vi "Dashboard Main.vi"() -> ()   [LabVIEW 2012]
uses:
  <vilib>/event_ctls.llb/eventvkey.ctl
  <vilib>/Utility/config.llb/Read Key (String).vi
  <vilib>/Utility/config.llb/Read Key (I32).vi
  <vilib>/Utility/config.llb/Write Key (String).vi
  <vilib>/Utility/config.llb/Write Key (I32).vi
  <vilib>/Utility/config.llb/NI_LVConfig.lvlib
panel:
  out "Battery Value":dbl(slide) scale=0.0..14.0 scale format="%#_2e"
  out "Battery":sgl(graph)
  in  "Camera Settings":T1={"Frate Rate"=30, "Compression"=30, "Size"=1} {"Frate Rate" scale=1.0..30.0; "Size" items=["640x480", "320x240", "160x120"]}
  out "Mode":T2(ring)=enum."Auto Disabled"
  out "Camera IP":string
  out "JS1 Z":dbl(slide) scale=-1.0..1.0 scale format="%#_2e"
  out "JS2 Z":dbl(slide) scale=-1.0..1.0 scale format="%#_2e"
  out "Joystick 1":cluster{"X":dbl, "Y":dbl}[](graph)
  out "Joystick 2":cluster{"X":dbl, "Y":dbl}[](graph)
  out "JS Buttons 1":T3
  out "JS Buttons 2":T3
  out "MotorSlide4":dbl(slide) scale=-1.0..1.0 scale format="%#_2e"
  out "MotorSlide3":dbl(slide) scale=-1.0..1.0 scale format="%#_2e"
  out "MotorSlide2":dbl(slide) scale=-1.0..1.0 scale format="%#_2e"
  in  "MotorName3":string="Front Left"
  in  "MotorName4":string="Front Right"
  in  "MotorName1":string="Rear Left"
  in  "MotorName2":string="Rear Right"
  out "MotorChart4":dbl(graph)
  out "MotorChart3":dbl(graph)
  out "MotorChart2":dbl(graph)
  out "MotorSlide1":dbl(slide) scale=-1.0..1.0 scale format="%#_2e"
  out "MotorChart1":dbl(graph)
  out "Robot IP":string
  in  "Dashboard Tab":enum32{"Operation", "Test", "Checklist"}(tab)
  in  "Drivetrain Position":dbl
  in  "Right Add":dbl
  in  "Left Add":dbl
  in  "Checkbox 2":bool
  in  "Checkbox 1":bool
  in  "Slider 1":dbl(slide) scale=0.0..100.0
  in  "Back Shooter Speed":dbl=1500.0
  in  "Front Shooter Speed":dbl=1500.0
  out "Back Shooter Feedback":dbl
  out "Front Shooter Feedback":dbl
  in  "Ball Screw Angle":dbl=0.5
  out "Ball Screw \nFeedback":dbl
  in  "Slider":dbl(slide) scale=0.0..100.0 scale format="%#_3g"
  in  "On/Off":bool caption="Solenoid"
  in  "Test Name":u16(ring) items=["Select the test to run...", "Example Test", "-------------------------------", "List of tests is built in robot code.", "Replace with your own automated tests."]
  in  "Test Tree":string(tree)
  in  "Motor":cluster{"Value":dbl, "Enable":bool} {"Value" scale=-1.0..1.0 scale format="%#_3g"}
  out "Progress":T4 {"Test Progress" scale=0.0..100.0}
  in  "Rev/Fwd":cluster{"Forward":bool, "Reverse":bool}
  in  "Ring":u16(ring) items=["Auto", "Fixed indoor", "Fixed outdoor 1", "Fixed outdoor 2", "Fixed fluorescent 1", "Fixed fluorescent 2", "Hold current"]
  in  "Listbox":i32(listbox)
  in  "Viewer":T5(tab)
  out "Mbps":dbl format="%#.1g"
  in  "Enable":bool
  in  "DB Camera Config":bool
  out "Mbps":bool
  out "fps":dbl format="%#.1g"
  out "Image Error Message":string="Timeout in Camera Communications"
  out "Camera Image":T6(plugin-control)
  out "Buttons 1":cluster{"1":bool, "2":bool, "3":bool}
  out "Kinect 1":cluster{"X":dbl, "Y":dbl, "Z":dbl} {"X" scale=1.0..-1.0; "Y" scale=1.0..-1.0; "Z" scale=1.0..-1.0}
  out "Buttons 2":cluster{"1":bool, "2":bool, "3":bool}
  out "Kinect 2":cluster{"X":dbl, "Y":dbl, "Z":dbl} {"X" scale=1.0..-1.0; "Y" scale=1.0..-1.0; "Z" scale=1.0..-1.0}
  out "Version":string
  out "Skeleton Picture":picture
  out "Players":i8
  out "Tree":string(tree)
  # "Drive & Motors"
  # "Robot IP:"
  # "Customize by placing controls and indicators here and name to match\nDashboard Variables on robot."
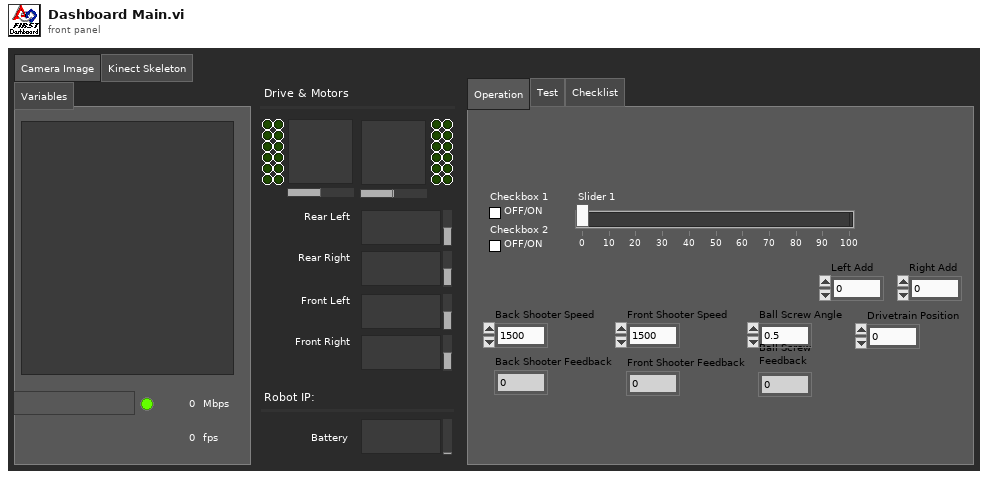
[diagram p1: front panel]
types:
  T1 = cluster{"Frate Rate":i32, "Compression":i32, "Size":u16}
  T2 = enum8{"Tele-Op Disabled", "Tele-Op Enabled", "Auto Disabled", "Auto Enabled", "Test Disabled", "Test Enabled", ""}
  T3 = cluster{bool, bool, bool, bool, bool, bool, bool, bool, bool, bool, bool, bool}
  T4 = cluster{"Test Progress":u8, "Test Progress Text":string}
  T5 = enum32{"Camera Image", "Kinect Skeleton", "Variables"}
  T6 = typedef "IMAQ Image.ctl" = refnum<image>
  T7 = typedef "Image Type" = u32
  T8 = typedef "LVBoundsTypeDef.ctl" = cluster{"Width":u32, "Height":u32}
  T9 = typedef "SkeletonTrackState.ctl" = enum32{"NotTracked", "PositionOnly", "Tracked"}
  T10 = cluster{"TrackingState":u8[], "Position":cluster{"x":sgl, "y":sgl, "z":sgl}, cluster{"x":sgl, "y":sgl, "z":sgl, sgl}[], "TrackState":T9}
  T11 = cluster{cluster{"ScaledToPercentRange":dbl, "ScaledToPercentRange":dbl, "ScaledToPercentRange":dbl}, cluster{bool, bool, bool}}[]
  T12 = cluster{cluster{"ScaledToPercentRange":dbl, "ScaledToPercentRange":dbl, "ScaledToPercentRange":dbl}, cluster{bool, bool, bool}}
  T13 = cluster{"ScaledToPercentRange":dbl, "ScaledToPercentRange":dbl, "ScaledToPercentRange":dbl}
  T14 = typedef "LVRectTypeDef.ctl" = cluster{"Left":i16, "Top":i16, "Right":i16, "Bottom":i16}
  T15 = cluster{"Competition mode":bool, "Robot Link":bool, "Autonomous":bool, "Enabled":bool, "E-Stop":bool, "Simulated":bool, "TestMode":bool, "Docked Window":bool}
  T16 = cluster{"Boolean Array[0]":bool, "Boolean Array[1]":bool, "Boolean Array[2]":bool, "Boolean Array[3]":bool, "Boolean Array[4]":bool, "Boolean Array[5]":bool, "Boolean Array[6]":bool, "Boolean Array[7]":bool, "Boolean Array[8]":bool, "Boolean Array[9]":bool, "Boolean Array[10]":bool, "Boolean Array[11]":bool}
  T17 = typedef "NI_LVConfig.lvlib/Config Data RefNum.ctl" = refnum<k1>
  T18 = typedef "eventvkey.ctl" = enum16{"ASCII", "Enter", "Return", "Shift", "Ctrl", "Alt", "Cmd", "Opt", "Caps", "NumLock", "Clear", "Break", "Up", "Down", "Left", "Right", "Insert", "Delete", "Home", "End", "PageUp", "PageDown", "Escape", "Help", "Pause", "ScrollLock", "F1", "F2", "F3", "F4", "F5", "F6", "F7", "F8", "F9", "F10", "F11", "F12", "F13", "F14", "F15", "F16", "F17", "F18", "F19", "F20", "F21", "F22", "F23", "F24", "Play", "VolumeUp", "VolumeDown", "Mute", "Two Byte Char"}
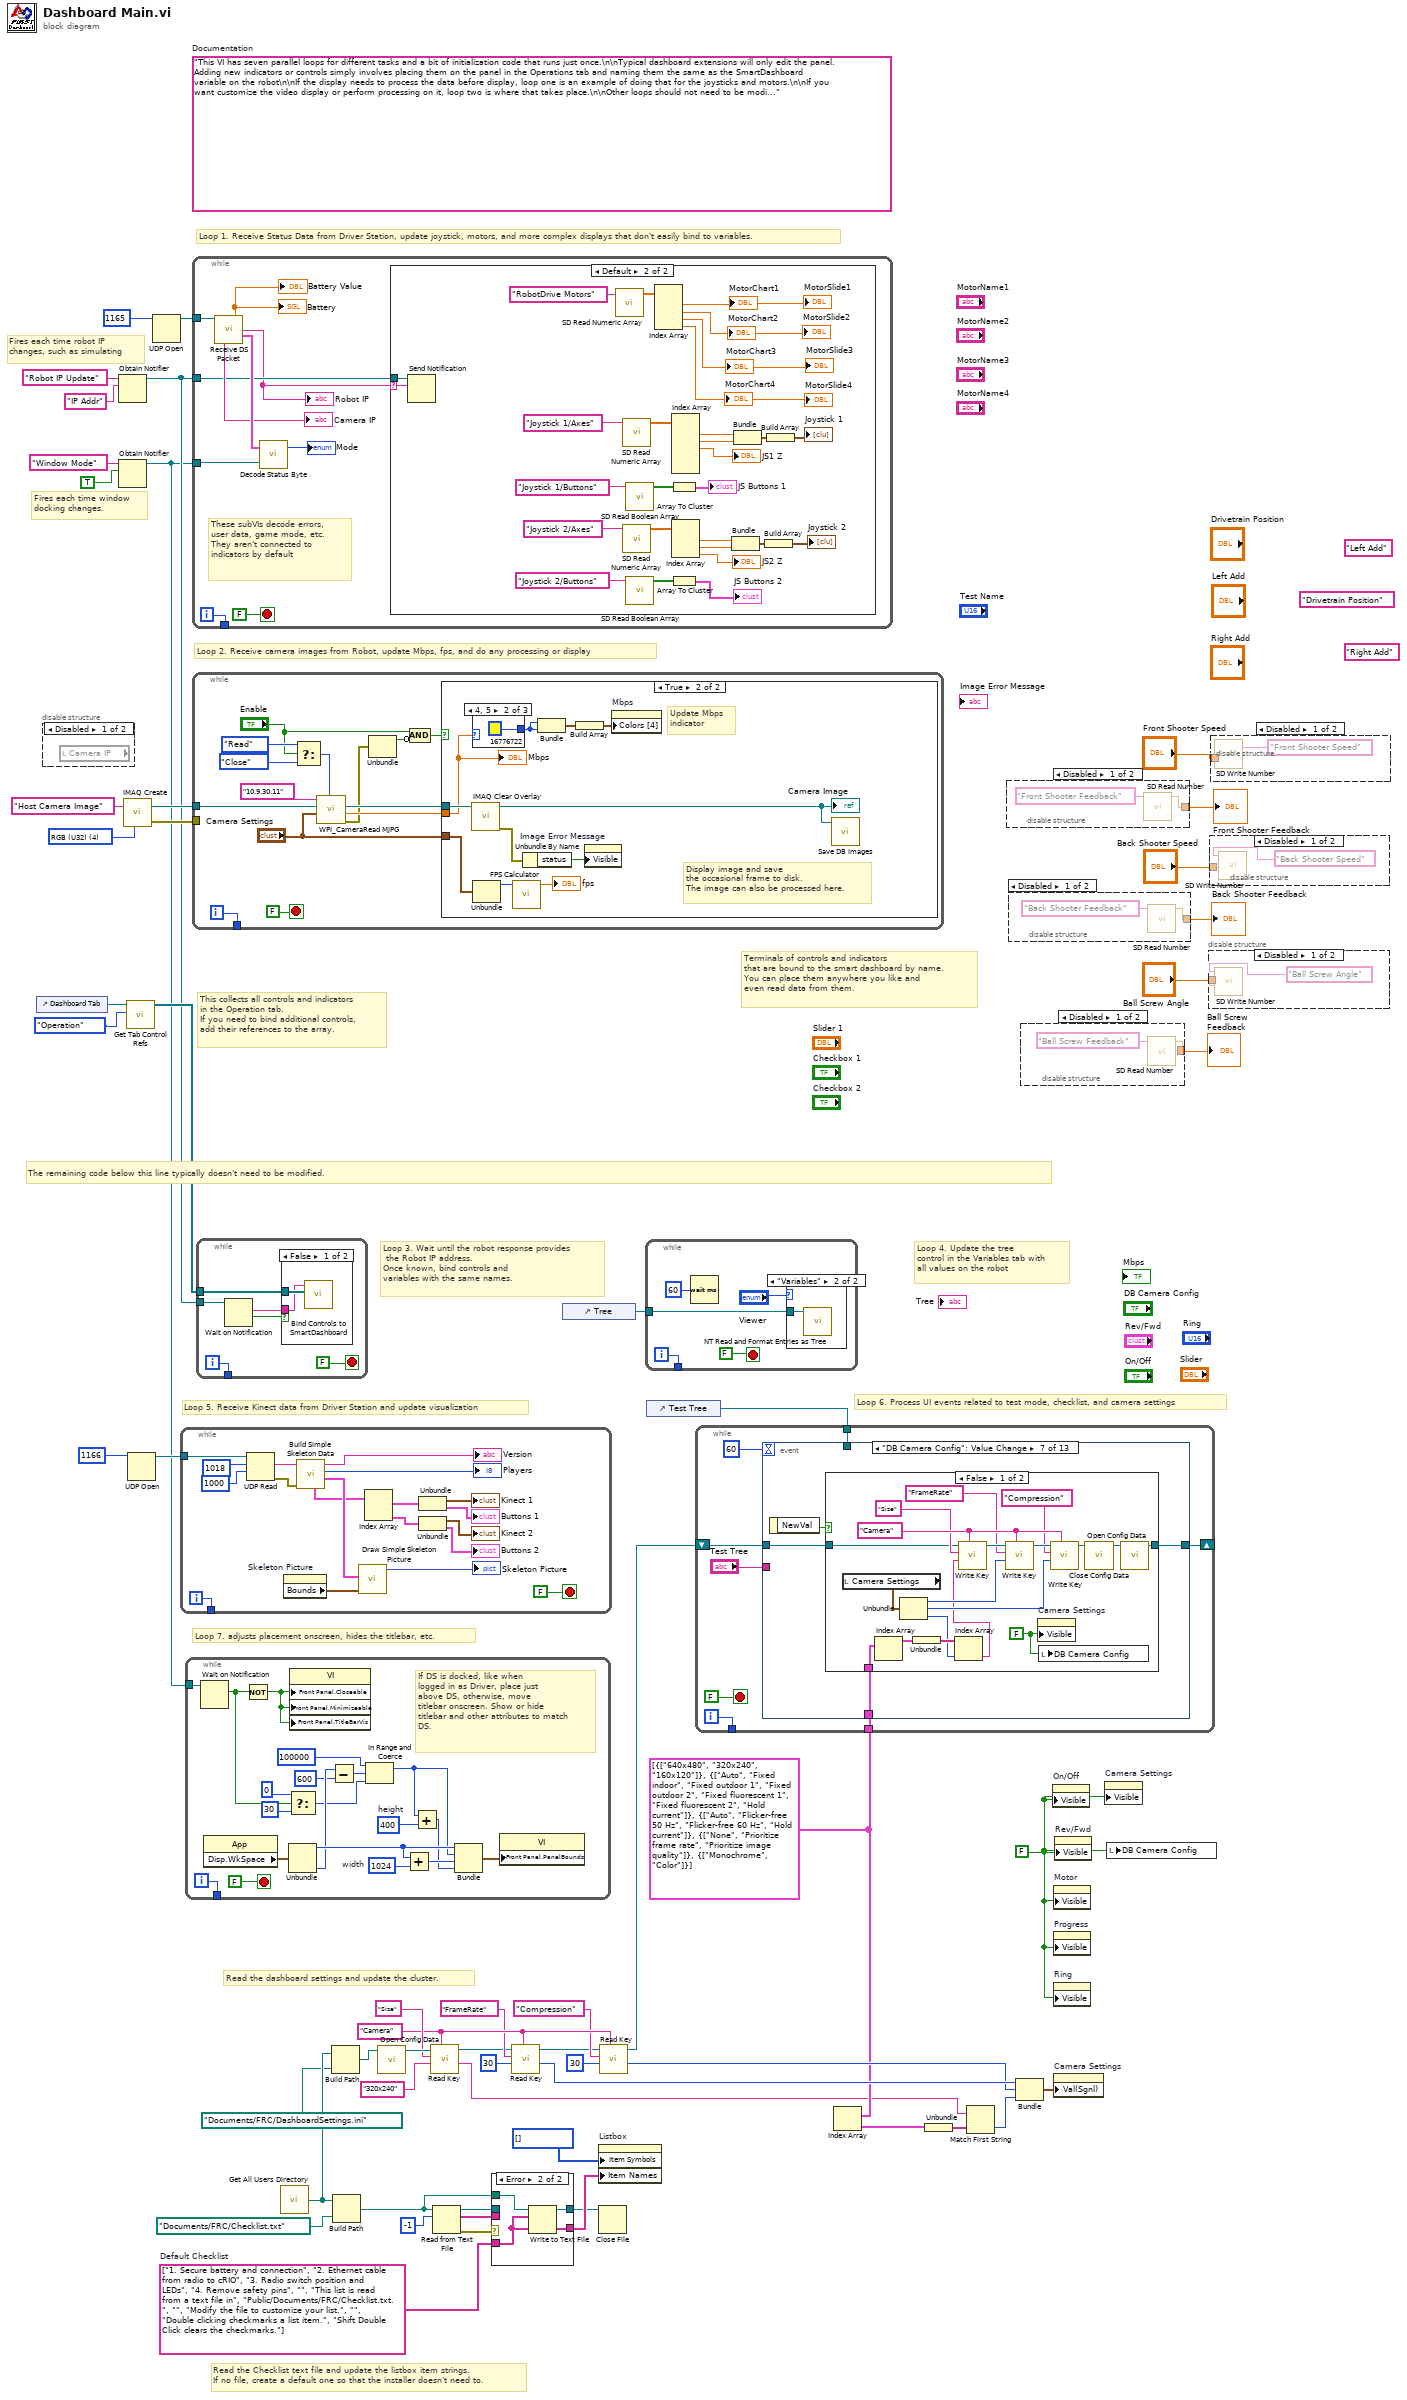
[diagram p0: block diagram]
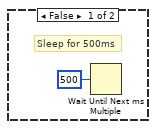
[diagram p10: hidden frame]
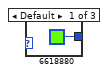
[diagram p11: hidden frame]
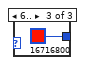
[diagram p12: hidden frame]
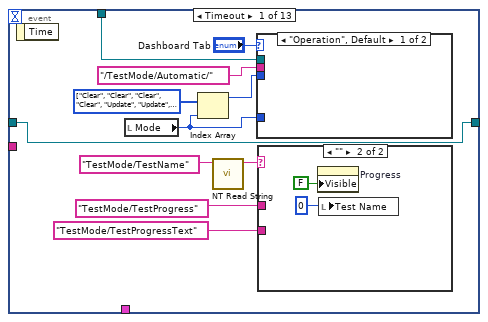
[diagram p14: hidden frame]
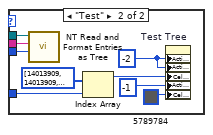
[diagram p15: hidden frame]
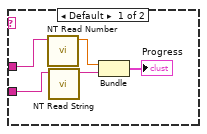
[diagram p16: hidden frame]
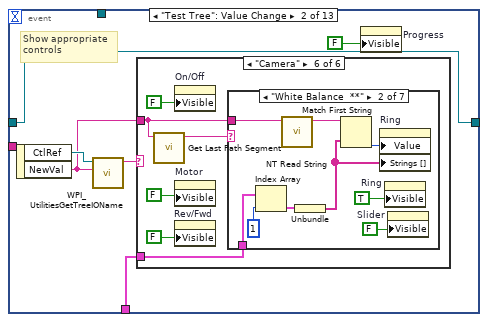
[diagram p17: hidden frame]
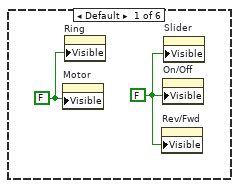
[diagram p18: hidden frame]
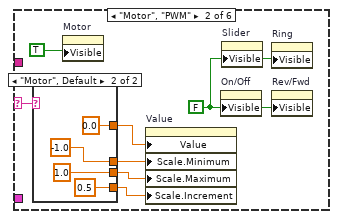
[diagram p19: hidden frame]
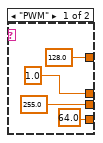
[diagram p20: hidden frame]
diagram:
  (unwired) "Right Add" ("Name")
  (unwired) "Left Add" ("Name")
  (unwired) "Drivetrain Position" ("Name")
  w27 = "Camera"
  w19 = cluster{string[]}[] [{["640x480", "320x240", "160x120"]}, {["Auto", "Fixed indoor", "Fixed outdoor 1", "Fixed outdoor 2", "Fixed fluorescent 1", "Fixed fluorescent 2", "Hold current"]}, {["Auto", "Flicker-free 50 Hz", "Flicker-free 60 Hz", "Hold current"]}, {["None", "Prioritize frame rate", "Prioritize image quality"]}, {["Monochrome", "Color"]}]
  w35 = string[] ["1. Secure battery and connection", "2. Ethernet cable from radio to cRIO", "3. Radio switch position and LEDs", "4. Remove safety pins", "", "This list is read from a text file in", "Public/Documents/FRC/Checklist.txt.", "", "Modify the file to customize your list.", "", "Double clicking checkmarks a list item.", "Shift Double Click clears the checkmarks."]  # Default Checklist
  w33 = FALSE ("Visible")
  (unwired) "This VI has seven parallel loops for different tasks and a bit of initialization code that runs just once.\n\nTypical dashboard extensions will only edit the panel. Adding new indicators or controls simply involves placing them on the panel in the Operations tab and naming them the same as the SmartDashboard variable on the robot\n\nIf the display needs to process the data before display, loop one is an example of doing that for the joysticks and motors.\n\nIf you want customize the video display or perform processing on it, loop two is where that takes place.\n\nOther loops should not need to be modified. They are pretty standard, and document the task they perform."  # Documentation
  w56 = T7 4 items=["Grayscale (U8)", "Grayscale (I16)", "Grayscale (SGL)", "Complex (CSG)", "RGB (U32)", "HSL (U32)", "RGB (U64)"] ("Image Type")
  # "Fires each time robot IP\nchanges, such as simulating"
  # "Fires each time window\ndocking changes."
  # "Read the Checklist text file and update the listbox item strings.\nIf no file, create a default one so that the installer doesn't need to."
  # "This collects all controls and indicators\nin the Operation tab.\nIf you need to bind additional controls,\nadd their references to the array."
  # "The remaining code below this line typically doesn't need to be modified."
  # "Loop 6. Process UI events related to test mode, checklist, and camera settings"
  # "Read the dashboard settings and update the cluster."
  # "Terminals of controls and indicators\nthat are bound to the smart dashboard by name.\nYou can place them anywhere you like and\neven read data from them."
  # "Loop 4. Update the tree\ncontrol in the Variables tab with\nall values on the robot"
  # "Loop 3. Wait until the robot response provides\n the Robot IP address.\nOnce known, bind controls and\nvariables with the same names."
  # "Loop 5. Receive Kinect data from Driver Station and update visualization"
  # "Loop 7. adjusts placement onscreen, hides the titlebar, etc."
  # "Loop 1. Receive Status Data from Driver Station, update joystick, motors, and more complex displays that don't easily bind to variables."
  # "Loop 2. Receive camera images from Robot, update Mbps, fps, and do any processing or display"
  n1 = control-ref of="Dashboard Tab"() -> (w49:refnum<vi>)
  n2 = disable-structure shown="Disabled" {
    frame Disabled {
      n3 = local read "Camera IP"() -> ()  [unwired: 1 out]
    }
    frame Enabled {
    }
  }
  n4 = Obtain Notifier(name (unnamed)="Robot IP Update", notification data type="IP Addr" ("name (unnamed)")) -> (notifier out=w46:refnum<notifier>)  [unwired: 2 in, 2 out]
  n5 = Obtain Notifier(name (unnamed)="Window Mode", notification data type=TRUE) -> (notifier out=w39:refnum<notifier>)  [unwired: 2 in, 2 out]
  n6 = call "IMAQ Create"("Image Name"="Host Camera Image", "Image Type"=w56) -> ("New Image"=w54:T6, "error out"=w53:errorcluster)  [unwired: 2 in, 1 out]
  n7 = call <vilib>:"Get Tab Control Refs.vi"("Page Index"=enum32{"Operation", "Test"}."Operation" ("Dashboard Tab"), "TabControl in"=w49) -> ("ControlsOnPage"=w50:refnum<vi>[])  [unwired: 9 in]
  n8 = UDP Open(11:u16 1166 ("port")) -> (port=w51:refnum<k16>)  [unwired: 2 in, 4 out]
  n9 = UDP Open(11:u16 1165 ("port")) -> (port=w57:refnum<k16>)  [unwired: 2 in, 4 out]
  n10 = while {
    tunnel: w51 -> [w75]
    tunnel: [w60] -> _
    i -> [w60]
    stop <- FALSE stop-if-true
    n11 = UDP Read(connection ID=w75, max size (548)=1018 ("bytes to read"), timeout ms (25000)=1000) -> (data out=w69:string, error out=w59:errorcluster)  [unwired: 1 in, 3 out]
    n12 = property on="Skeleton Picture" class="Pict"() -> ("Bounds"=w71:T8)  [unwired: 2 in, 2 out]
    n13 = call "Build Simple Skeleton Data.vi"("error in (no error)"=w59, "data in"=w69) -> ("Skeleton Data"=w70:T10, "NumPlayers"=→"Players":i8, "Version String"=→"Version":string, "Simple Joystick Info"=w67:T11)  [unwired: 5 in, 1 out]
    n14 = call "Draw Simple Skeleton Picture.vi"("Bounds"=w71, "Simple Skeleton"=w70) -> ("new picture out"=→"Skeleton Picture":picture)  [unwired: 9 in]
    n15 = Index Array(array=w67) -> (element #1=w66:T12, element #2=w65:T12)  [unwired: 2 in]
    n16 = Unbundle(w66) -> (→"Kinect 1":T13, →"Buttons 1":cluster{bool, bool, bool})
    n17 = Unbundle(w65) -> (→"Kinect 2":T13, →"Buttons 2":cluster{bool, bool, bool})
  }
  n18 = while {
    tunnel: w39 -> [w96]
    tunnel: [w94] -> _
    i -> [w94]
    stop <- FALSE stop-if-true
    w86 = 1024  # width
    w89 = 400  # height
    # "If DS is docked, like when\nlogged in as Driver, place just\nabove DS, otherwise, move\ntitlebar onscreen. Show or hide\ntitlebar and other attributes to match\nDS."
    n19 = Wait on Notification(notifier=w96) -> (notification=w81:bool)  [unwired: 3 in, 3 out]
    n20 = property class="App"() -> ("Disp.WkSpace"=w92:T14)  [unwired: 2 in, 2 out]
    n21 = Not(x=w81) -> (.not. x?=w95:bool)
    n22 = Unbundle(w92) -> ("Left"=w90:i16, "Bottom"=w87:i16)  [unwired: 2 out]
    n23 = Select(t=0, s=w81, f=30) -> (s? t:f=w80:i32)
    n24 = property class="VI"("Front Panel.Closeable"=w95, "Front Panel.Minimizeable"=w95, "Front Panel.TitleBarVis"=w95) -> ()  [unwired: 2 in, 2 out]
    n25 = Subtract(x=w87, y=600) -> (x-y=w84:i32)
    n26 = In Range and Coerce(upper limit=100000, x=w84, lower limit=w80) -> (coerced(x)=w78:i32)  [unwired: 1 out]
    n27 = Add(x=w90, y=w86) -> (x+y=w91:i32)
    n28 = Add(x=w78, y=w89) -> (x+y=w88:i32)
    n29 = Bundle("Left"=w90, w78, w91, w88) -> (w93:cluster{"Left":i16, i32, i32, i32})  [unwired: 1 out]
    n30 = property class="VI"("Front Panel.PanelBounds"=w93) -> ()  [unwired: 2 in, 2 out]
  }
  n31 = while {
    tunnel: w54 -> [w108]
    tunnel: w53 -> [_]
    tunnel: [w110] -> _
    i -> [w110]
    stop <- FALSE stop-if-true
    n32 = Select(t=enum16{"Read", "Reopen", "Close"}."Read" ("Operation"), s="Enable", f=enum16{"Read", "Reopen", "Close"}."Close" ("Operation")) -> (s? t:f=w103:enum16{"Read", "Reopen", "Close"})
    n33 = call <vilib>:"WPI_CameraRead MJPG.vi"("Operation"=w103, "Camera Settings"="Camera Settings", "Image"=w108, "address"="10.9.30.11") -> ("error out"=w102:errorcluster, "Bandwidth (kbps)"=w106:dbl, "Image Out"=w107:T6)  [unwired: 5 in]
    n34 = Unbundle(w102) -> ("status"=w100:bool)  [unwired: 2 out]
    n35 = Compound Arithmetic op=AND("Enable", invert w100) -> (w99:bool)
    n36 = case shown="True" w99 {
      tunnel: "Camera Settings" -> [_ w114]
      tunnel: w107 -> [_ w117]
      tunnel: w106 -> [_ w116]
      frame False {
        # "Sleep for 500ms"
        n37 = Wait Until Next ms Multiple(millisecond multiple=u32 500) -> ()  [unwired: 1 out]
      }
      frame True {
        # "Display image and save\nthe occasional frame to disk.\nThe image can also be processed here."
        # "Update Mbps\nindicator"
        n38 = call "IMAQ Clear Overlay"("Image"=w117) -> ("error out"=w122:errorcluster, "Image Out"=w121:T6)  [unwired: 2 in, 7 out]
        "Camera Image" <- w121
        n39 = case shown="4, 5" w116 {
          tunnel: [u32 6618880 ("Color Box") u32 16776722 ("Color Box") u32 16716800 ("Color Box")] -> w118
          frame Default {
          }
          frame 4, 5 {
          }
          frame 6.. {
          }
        }
        n40 = Unbundle(w114) -> ("Frate Rate"=w113:i32)  [unwired: 2 out]
        n41 = call "FPS Calculator.vi"("Average Count"=w113) -> ("fps"=→"fps":dbl)  [unwired: 10 in]
        n42 = Unbundle By Name(w122) -> ("status"=w123:bool)
        n43 = Bundle("Color Box"=w118, "Color Box"=w118) -> (w120:cluster{"Color Box":u32, "Color Box":u32})  [unwired: 1 out]
        n44 = Build Array(w120) -> (w119:cluster{"Color Box":u32, "Color Box":u32}[])
        n45 = property on="Image Error Message" class="Str"("Visible"=w123) -> ()  [unwired: 2 in, 2 out]
        n46 = property on="Mbps" class="Bool (strict)"("Colors [4]"=w119) -> ()  [unwired: 2 in, 2 out]
        n47 = call "Save DB Images.vi"("Image"=w121) -> ()  [unwired: 2 in, 1 out]
        "Mbps" <- w116
      }
    }
  }
  n48 = while {
    tunnel: w57 -> [w134]
    tunnel: w46 -> [w128]
    tunnel: w39 -> [w132]
    tunnel: [w129] -> _
    i -> [w129]
    stop <- FALSE stop-if-true
    # "These subVIs decode errors, user data, game mode, etc.\nThey aren't connected to indicators by default"
    n49 = call "Receive DS Packet.vi"("Recv Socket"=w134) -> ("Battery"=→"Battery" →"Battery Value":sgl, "Robot IP Address"=w127:string, "Status"=w135:T15, "Camera IP Address"=→"Camera IP":string)  [unwired: 1 in, 10 out]
    "Robot IP" <- w127
    n50 = call "Decode Status Byte.vi"("Window Mode Notifier"=w132, "Status"=w135) -> ("Mode"=→"Mode":T2)  [unwired: 1 out]
    n51 = case shown="Default" w127 {
      selector: w127 -> [_ w137]
      tunnel: w128 -> [_ w138]
      frame "0.0.0.0" {
        # "Robot not responding, don't poll the variables"
      }
      frame Default {
        n52 = Send Notification(notification=w137, notifier=w138) -> ()  [unwired: 1 in, 2 out]
        n53 = call <vilib>:"SD Read Numeric Array.vi"("Name"="RobotDrive Motors") -> ("Numeric Array"=w161:dbl[])  [unwired: 8 in, 2 out]
        n54 = call <vilib>:"SD Read Numeric Array.vi"("Name"="Joystick 1/Axes") -> ("Numeric Array"=w154:dbl[])  [unwired: 8 in, 2 out]
        n55 = call <vilib>:"SD Read Numeric Array.vi"("Name"="Joystick 2/Axes") -> ("Numeric Array"=w148:dbl[])  [unwired: 8 in, 2 out]
        n56 = call <vilib>:"SD Read Boolean Array.vi"("Name"="Joystick 1/Buttons") -> ("Boolean Array"=w156:bool[])  [unwired: 8 in, 2 out]
        n57 = call <vilib>:"SD Read Boolean Array.vi"("Name"="Joystick 2/Buttons") -> ("Boolean Array"=w147:bool[])  [unwired: 8 in, 2 out]
        n58 = Index Array(array=w161) -> (element #1=→"MotorChart1" →"MotorSlide1":dbl, element #2=→"MotorSlide2" →"MotorChart2":dbl, element #3=→"MotorChart3" →"MotorSlide3":dbl, element #4=→"MotorChart4" →"MotorSlide4":dbl)  [unwired: 4 in]
        n59 = Array To Cluster(array=w156) -> (cluster=→"JS Buttons 1":T16)
        n60 = Array To Cluster(array=w147) -> (cluster=→"JS Buttons 2":T16)
        n61 = Index Array(array=w154) -> (element #1=w151:dbl, element #2=w152:dbl, element #3=→"JS1 Z":dbl)  [unwired: 6 in, 3 out]
        n62 = Index Array(array=w148) -> (element #1=w143:dbl, element #2=w142:dbl, element #3=→"JS2 Z":dbl)  [unwired: 3 in]
        n63 = Bundle("Numeric"=w143, "Numeric"=w142) -> (w144:cluster{"Numeric":dbl, "Numeric":dbl})  [unwired: 1 in]
        n64 = Bundle("Numeric"=w151, "Numeric"=w152) -> (w150:cluster{"Numeric":dbl, "Numeric":dbl})  [unwired: 1 in]
        n65 = Build Array(w144) -> (→"Joystick 2":cluster{"Numeric":dbl, "Numeric":dbl}[])
        n66 = Build Array(w150) -> (→"Joystick 1":cluster{"Numeric":dbl, "Numeric":dbl}[])
      }
    }
  }
  n67 = while {
    tunnel: w50 -> [w170]
    tunnel: w46 -> [w167]
    tunnel: [w165] -> _
    i -> [w165]
    stop <- FALSE stop-if-true
    n68 = Wait on Notification(notifier=w167) -> (notification=w166:string, timed out?=w168:bool)  [unwired: 3 in, 2 out]
    n69 = case shown="False" w168 {
      tunnel: w170 -> [w172 _]
      tunnel: w166 -> [w171 _]
      frame False {
        n70 = call <vilib>:"Bind Controls to SmartDashboard.vi"("Bound Control Refs"=w172, "Server IP Address"=w171) -> ()  [unwired: 10 in]
      }
      frame True {
      }
    }
  }
  n71 = call "Get All Users Directory.vi"() -> ("All User Path"=w32:path)
  n72 = Build Path(base path=w32, name or relative path=path "Documents/FRC/DashboardSettings.ini") -> (appended path=w31:path)
  n73 = Build Path(base path=w32, name or relative path=path "Documents/FRC/Checklist.txt") -> (appended path=w36:path)
  n74 = call <vilib>:"Open Config Data.vi"("configuration file path"=w31) -> ("refnum"=w30:T17)  [unwired: 8 in, 2 out]
  n75 = call-poly <vilib>:"Read Key.vi"("section"=w27, "default value"="320x240", "key"="Size", "refnum"=w30) -> ("value"=w17:string, "refnum out"=w12:T17)  [unwired: 2 in, 4 out]
  n76 = Read from Text File(file (use dialog)=w36, count=-1 ("timeout ms (25000)")) -> (refnum out=w14:refnum<file>, text=w37:string[], error out=w38:errorcluster)  [unwired: 2 in, 1 out]
  n77 = case shown="Error" w38 {
    tunnel: w37 -> [w174 _]
    tunnel: [w174 w176] -> w34
    tunnel: w35 -> [_ w176]
    tunnel: w36 -> [_ w177]
    tunnel: [w173 w175] -> w13
    tunnel: w14 -> [w173 _]
    frame No Error {
    }
    frame Error {
      n78 = Write to Text File(file (use dialog)=w177, text=w176) -> (refnum out=w175:refnum<file>)  [unwired: 2 in, 2 out]
    }
  }
  n79 = call-poly <vilib>:"Read Key.vi"("section"=w27, "default value"=30, "key"="FrameRate", "refnum"=w12) -> ("value"=w22:i32, "refnum out"=w11:T17)  [unwired: 1 in, 5 out]
  n80 = control-ref of="Tree"() -> (w8:refnum<vi>)
  n81 = property on="Listbox" class="LstBox (strict)"("Item Symbols"=i32[] [], "Item Names"=w34) -> ()  [unwired: 2 in, 2 out]
  n82 = Close File(refnum=w13) -> ()  [unwired: 1 in, 2 out]
  n83 = call-poly <vilib>:"Read Key.vi"("section"=w27, "default value"=30, "key"="Compression", "refnum"=w11) -> ("value"=w21:i32, "refnum out"=w9:T17)  [unwired: 1 in, 5 out]
  n84 = while {
    tunnel: [w179] -> _
    tunnel: w8 -> [w178]
    i -> [w179]
    stop <- FALSE stop-if-true
    n85 = Wait (ms)(milliseconds to wait=u32 60) -> ()  [unwired: 1 out]
    n86 = case shown="\"Variables\"" "Viewer" {
      tunnel: w178 -> [_ w183]
      frame Default {
      }
      frame "Variables" {
        n87 = call <vilib>:"NT Read and Format Entries as Tree.vi"("Tree Refnum"=w183) -> ()  [unwired: 9 in, 2 out]
      }
    }
  }
  n88 = control-ref of="Test Tree"() -> (w7:refnum<vi>)
  n89 = while {
    tunnel: w19 -> [w188]
    shift-right: [w187] -> _
    shift-left: w9 -> [w186]
    tunnel: [w185] -> _
    tunnel: w7 -> [w184]
    i -> [w185]
    stop <- FALSE stop-if-true
    n90 = event shown="[6] \"DB Camera Config\": Value Change" {
      selector: _ -> [_ _ _ _ _ _ _ _ _ _ _ _ _]
      dyn-events: _ -> [_ _ _ _ _ _ _ _ _ _ _ _ _]
      timeout: u32 60 ("milliseconds to wait") -> [_ _ _ _ _ _ _ _ _ _ _ _ _]
      tunnel: w184 -> [w198 _ _ _ _ _ _ _ _ _ _ _ _]
      tunnel: "Test Tree" -> [_ _ _ _ _ _ _ _ w392 w400 w402 w406 w414]
      tunnel: w188 -> [_ w220 _ _ _ _ w356 w386 _ _ _ _ _]
      tunnel: [w192 w219 _ w322 w330 w342 w355 w379 w391 w398 w401 w405 w413] -> w187
      tunnel: w186 -> [w192 w219 _ w322 w330 w342 w354 w379 w391 w398 w401 w405 w413]
      event Timeout {
        w197 = enum16{"Update", "Clear"}[] [enum."Clear", enum."Clear", enum."Clear", enum."Clear", enum."Update", enum."Update", enum."Clear"] items=["Update", "Clear"]
        n91 = event-data() -> ()  [unwired: 1 in, 1 out]
        n92 = local read "Mode"() -> (w195:T2)
        n93 = Index Array(array=w197, index=w195) -> (element=w196:enum16{"Update", "Clear"})
        n94 = call <vilib>:"NT Read String.vi"("Name"="TestMode/TestName") -> ("String"=w201:string)  [unwired: 9 in, 1 out]
        n95 = case shown="\"Operation\", Default" "Dashboard Tab" {
          tunnel: w198 -> [_ w211]
          tunnel: "/TestMode/Automatic/" ("Name Pattern") -> [_ w210]
          tunnel: w196 -> [_ w209]
          tunnel: w195 -> [_ w207]
          frame "Operation", Default {
          }
          frame "Test" {
            w206 = -2 ("Active Item:Row Number")
            n96 = call <vilib>:"NT Read and Format Entries as Tree.vi"("Operation"=w209, "Name Pattern"=w210, "Tree Refnum"=w211) -> ()  [unwired: 7 in, 2 out]
            n97 = Index Array(array=u32[] [14013909, 14013909, 14013909, 14013909, 14013909, 16777215, 14013909], index=w207) -> (element=w205:u32)
            n98 = property on="Test Tree" class="Tree (strict)"("Active Item Row Number"=w206, "ActiveColNum"=w206, "CellBG"=w205, "Active Item Row Number"=-1 ("Active Item:Row Number"), "CellBG"=u32 5789784 ("Color Box")) -> ()  [unwired: 2 in, 2 out]
          }
        }
        n99 = case shown="\"\"" w201 {
          tunnel: "TestMode/TestProgress" ("Name") -> [w213 _]
          tunnel: "TestMode/TestProgressText" ("Name") -> [w212 _]
          frame Default {
            n100 = call <vilib>:"NT Read Number.vi"("Name"=w213) -> ("Numeric"=w214:dbl)  [unwired: 9 in, 1 out]
            n101 = call <vilib>:"NT Read String.vi"("Name"=w212) -> ("String"=w215:string)  [unwired: 9 in, 1 out]
            n102 = Bundle("Numeric"=w214, "String"=w215) -> (→"Progress":cluster{"Numeric":dbl, "String":string})  [unwired: 1 in]
          }
          frame "" {
            n103 = property on="Progress" class="Clust (strict)"("Visible"=FALSE) -> ()  [unwired: 2 in, 2 out]
            n104 = local write "Test Name"(u16 0) -> ()
          }
        }
      }
      event "Test Tree": Value Change {
        # "Show appropriate\ncontrols"
        n105 = event-data() -> ("CtlRef"=w223:refnum<vi>, "NewVal"=w221:string)  [unwired: 1 in]
        n106 = call <vilib>:"WPI_UtilitiesGetTreeIOName.vi"("NewVal"=w221, "TreeControl in"=w223) -> ("I/O Name"=w224:string)  [unwired: 9 in]
        n107 = case shown="\"Camera\"" w224 {
          selector: w224 -> [_ w231 _ w249 w258 _]
          tunnel: w221 -> [_ _ w246 w248 _ w265]
          tunnel: w220 -> [_ _ _ _ _ w264]
          frame Default {
            w226 = FALSE ("Visible")
            w225 = FALSE ("Visible")
            n108 = property on="Motor" class="Clust (strict)"("Visible"=w225) -> ()  [unwired: 2 in, 2 out]
            n109 = property on="Ring" class="Ring (strict)"("Visible"=w225) -> ()  [unwired: 2 in, 2 out]
            n110 = property on="Rev/Fwd" class="Clust (strict)"("Visible"=w226) -> ()  [unwired: 2 in, 2 out]
            n111 = property on="On/Off" class="Bool (strict)"("Visible"=w226) -> ()  [unwired: 2 in, 2 out]
            n112 = property on="Slider" class="Slide (strict)"("Visible"=w226) -> ()  [unwired: 2 in, 2 out]
          }
          frame "Motor", "PWM" {
            w232 = FALSE ("Visible")
            n113 = case shown="\"Motor\", Default" w231 {
              tunnel: [1.0 ("Value") -1.0 ("Value")] -> w230
              tunnel: [255.0 ("Value") 1.0 ("Value")] -> w229
              tunnel: [128.0 ("Value") 0.0 ("Value")] -> w228
              tunnel: [64.0 ("Value") 0.5 ("Value")] -> w227
              frame "PWM" {
              }
              frame "Motor", Default {
              }
            }
            n114 = property on="Motor" class="Clust (strict)"("Visible"=TRUE) -> ()  [unwired: 2 in, 2 out]
            n115 = property on="Value" class="Slide (strict)"("Value"=w228, "Scale.Minimum"=w230, "Scale.Maximum"=w229, "Scale.Increment"=w227) -> ()  [unwired: 2 in, 2 out]
            n116 = property on="On/Off" class="Bool (strict)"("Visible"=w232) -> ()  [unwired: 2 in, 2 out]
            n117 = property on="Slider" class="Slide (strict)"("Visible"=w232) -> ()  [unwired: 2 in, 2 out]
            n118 = property on="Ring" class="Ring (strict)"("Visible"=w232) -> ()  [unwired: 2 in, 2 out]
            n119 = property on="Rev/Fwd" class="Clust (strict)"("Visible"=w232) -> ()  [unwired: 2 in, 2 out]
          }
          frame "Servo" {
            w244 = FALSE ("Visible")
            n120 = call <vilib>:"NT Read Number.vi"("Name"=w246) -> ("Numeric"=w245:dbl)  [unwired: 9 in, 1 out]
            n121 = property on="Slider" class="Slide (strict)"("Visible"=TRUE, "Scale.Maximum"=170.0 ("Scale.Range:Maximum")) -> ()  [unwired: 2 in, 2 out]
            n122 = local write "Slider"(w245) -> ()
            n123 = property on="Motor" class="Clust (strict)"("Visible"=w244) -> ()  [unwired: 2 in, 2 out]
            n124 = property on="Rev/Fwd" class="Clust (strict)"("Visible"=w244) -> ()  [unwired: 2 in, 2 out]
            n125 = property on="On/Off" class="Bool (strict)"("Visible"=w244) -> ()  [unwired: 2 in, 2 out]
            n126 = property on="Ring" class="Ring (strict)"("Visible"=w244) -> ()  [unwired: 2 in, 2 out]
          }
          frame "Relay", "Solenoid" {
            w247 = FALSE ("Visible")
            n127 = property on="Motor" class="Clust (strict)"("Visible"=w247) -> ()  [unwired: 2 in, 2 out]
            n128 = property on="Slider" class="Slide (strict)"("Visible"=w247) -> ()  [unwired: 2 in, 2 out]
            n129 = Search and Replace String(input string=w248, search string="/Value  **", replace string="/Direction") -> (result string=w254:string)  [unwired: 5 in, 3 out]
            n130 = property on="Ring" class="Ring (strict)"("Visible"=w247) -> ()  [unwired: 2 in, 2 out]
            n131 = call <vilib>:"NT Read String.vi"("Name"=w254) -> ("String"=w252:string)  [unwired: 9 in, 1 out]
            n132 = Equal?(x="Both directions", y=w252) -> (x = y?=w250:bool)
            n133 = Not(x=w250) -> (.not. x?=w251:bool)
            n134 = property on="Rev/Fwd" class="Clust (strict)"("Visible"=w250) -> ()  [unwired: 2 in, 2 out]
            n135 = property on="On/Off" class="Bool (strict)"("Visible"=w251, "Caption.Text"=w249) -> ()  [unwired: 2 in, 2 out]
          }
          frame "Compressor", "Digital Out" {
            w257 = FALSE ("Visible")
            # "Get direction and finish"
            n136 = property on="Motor" class="Clust (strict)"("Visible"=w257) -> ()  [unwired: 2 in, 2 out]
            n137 = property on="Slider" class="Slide (strict)"("Visible"=w257) -> ()  [unwired: 2 in, 2 out]
            n138 = property on="Ring" class="Ring (strict)"("Visible"=w257) -> ()  [unwired: 2 in, 2 out]
            n139 = property on="On/Off" class="Bool (strict)"("Visible"=TRUE, "Caption.Text"=w258) -> ()  [unwired: 2 in, 2 out]
            n140 = property on="Rev/Fwd" class="Clust (strict)"("Visible"=FALSE) -> ()  [unwired: 2 in, 2 out]
          }
          frame "Camera" {
            n141 = call <vilib>:"Get Last Path Segment.vi"("String in"=w265) -> ("String out"=w266:string)  [unwired: 10 in]
            n142 = property on="On/Off" class="Bool (strict)"("Visible"=FALSE) -> ()  [unwired: 2 in, 2 out]
            n143 = property on="Motor" class="Clust (strict)"("Visible"=FALSE) -> ()  [unwired: 2 in, 2 out]
            n144 = property on="Rev/Fwd" class="Clust (strict)"("Visible"=FALSE) -> ()  [unwired: 2 in, 2 out]
            n145 = case shown="\"White Balance  **\"" w266 {
              tunnel: w265 -> [w272 w281 w290 w299 w308 _ w314]
              tunnel: w264 -> [w270 w278 w287 w296 w305 _ _]
              frame "Size  **" {
                n146 = Index Array(array=w270) -> (element=w269:cluster{string[]})  [unwired: 1 in]
                n147 = call <vilib>:"NT Read String.vi"("Name"=w272) -> ("String"=w271:string)  [unwired: 9 in, 1 out]
                n148 = Unbundle(w269) -> (w267:string[])
                n149 = Match First String(2:w267, 3:w271) -> (0:w268:i32)  [unwired: 1 out]
                n150 = property on="Ring" class="Ring (strict)"("Value"=w268, "Strings []"=w267) -> ()  [unwired: 2 in, 2 out]
                n151 = property on="Ring" class="Ring (strict)"("Visible"=TRUE) -> ()  [unwired: 2 in, 2 out]
                n152 = property on="Slider" class="Slide (strict)"("Visible"=FALSE) -> ()  [unwired: 2 in, 2 out]
              }
              frame "White Balance  **" {
                n153 = Index Array(array=w278, index=1) -> (element=w279:cluster{string[]})
                n154 = call <vilib>:"NT Read String.vi"("Name"=w281) -> ("String"=w280:string)  [unwired: 9 in, 1 out]
                n155 = Unbundle(w279) -> (w276:string[])
                n156 = Match First String(2:w276, 3:w280) -> (0:w275:i32)  [unwired: 1 out]
                n157 = property on="Ring" class="Ring (strict)"("Value"=w275, "Strings []"=w276) -> ()  [unwired: 2 in, 2 out]
                n158 = property on="Ring" class="Ring (strict)"("Visible"=TRUE) -> ()  [unwired: 2 in, 2 out]
                n159 = property on="Slider" class="Slide (strict)"("Visible"=FALSE) -> ()  [unwired: 2 in, 2 out]
              }
              frame "Exposure  **" {
                n160 = Index Array(array=w287, index=2) -> (element=w288:cluster{string[]})
                n161 = call <vilib>:"NT Read String.vi"("Name"=w290) -> ("String"=w289:string)  [unwired: 9 in, 1 out]
                n162 = Unbundle(w288) -> (w284:string[])
                n163 = Match First String(2:w284, 3:w289) -> (0:w285:i32)  [unwired: 1 out]
                n164 = property on="Ring" class="Ring (strict)"("Value"=w285, "Strings []"=w284) -> ()  [unwired: 2 in, 2 out]
                n165 = property on="Ring" class="Ring (strict)"("Visible"=TRUE) -> ()  [unwired: 2 in, 2 out]
                n166 = property on="Slider" class="Slide (strict)"("Visible"=FALSE) -> ()  [unwired: 2 in, 2 out]
              }
              frame "Exposure Priority  **" {
                n167 = Index Array(array=w296, index=3) -> (element=w297:cluster{string[]})
                n168 = call <vilib>:"NT Read String.vi"("Name"=w299) -> ("String"=w298:string)  [unwired: 9 in, 1 out]
                n169 = Unbundle(w297) -> (w293:string[])
                n170 = Match First String(2:w293, 3:w298) -> (0:w294:i32)  [unwired: 1 out]
                n171 = property on="Ring" class="Ring (strict)"("Value"=w294, "Strings []"=w293) -> ()  [unwired: 2 in, 2 out]
                n172 = property on="Ring" class="Ring (strict)"("Visible"=TRUE) -> ()  [unwired: 2 in, 2 out]
                n173 = property on="Slider" class="Slide (strict)"("Visible"=FALSE) -> ()  [unwired: 2 in, 2 out]
              }
              frame "Color Enable  **" {
                n174 = Index Array(array=w305, index=4) -> (element=w306:cluster{string[]})
                n175 = call <vilib>:"NT Read String.vi"("Name"=w308) -> ("String"=w307:string)  [unwired: 9 in, 1 out]
                n176 = Unbundle(w306) -> (w302:string[])
                n177 = Match First String(2:w302, 3:w307) -> (0:w303:i32)  [unwired: 1 out]
                n178 = property on="Ring" class="Ring (strict)"("Value"=w303, "Strings []"=w302) -> ()  [unwired: 2 in, 2 out]
                n179 = property on="Ring" class="Ring (strict)"("Visible"=TRUE) -> ()  [unwired: 2 in, 2 out]
                n180 = property on="Slider" class="Slide (strict)"("Visible"=FALSE) -> ()  [unwired: 2 in, 2 out]
              }
              frame Default {
                n181 = property on="Ring" class="Ring (strict)"("Visible"=FALSE) -> ()  [unwired: 2 in, 2 out]
                n182 = property on="Slider" class="Slide (strict)"("Visible"=FALSE) -> ()  [unwired: 2 in, 2 out]
              }
              frame "Brightness  **", "Color Level  **", "Compression  **", "FPS  **", "Sharpness  **" {
                n183 = call <vilib>:"NT Read Number.vi"("Name"=w314) -> ("Numeric"=w313:dbl)  [unwired: 9 in, 1 out]
                n184 = local write "Slider"(w313) -> ()
                n185 = property on="Slider" class="Slide (strict)"("Visible"=TRUE, "Scale.Maximum"=100.0 ("Scale.Range:Maximum")) -> ()  [unwired: 2 in, 2 out]
                n186 = property on="Ring" class="Ring (strict)"("Visible"=FALSE) -> ()  [unwired: 2 in, 2 out]
              }
            }
          }
        }
        n187 = property on="Progress" class="Clust (strict)"("Visible"=FALSE) -> ()  [unwired: 2 in, 2 out]
      }
      event "Test Name": Mouse Enter {
        # "Populate the ring with the list of tests"
        n188 = event-data() -> ()  [unwired: 1 in, 1 out]
        n189 = call <vilib>:"NT Read String Array.vi"("Name"="TestMode/TestList") -> ("String Array"=w321:string[])  [unwired: 9 in, 1 out]
        n190 = Build Array (concatenate)("Select the test to run...", w321) -> (w320:string[])
        n191 = property on="Test Name" class="Ring (strict)"("Strings []"=w320) -> ()  [unwired: 2 in, 2 out]
      }
      event "Test Name": Value Change {
        w323 = FALSE ("Visible")
        # "Tell the robot the test name to run"
        n192 = event-data() -> ("NewVal"=w327:u16)  [unwired: 1 in]
        n193 = property on="Test Name" class="Ring (strict)"() -> ("Strings []"=w328:string[])  [unwired: 2 in, 2 out]
        n194 = local write "Progress"(T4 {"Test Progress"=0, "Test Progress Text"=""} ("Progress")) -> ()
        n195 = Index Array(array=w328, index=w327) -> (element=w326:string)
        n196 = call <vilib>:"NT Write String.vi"("String"=w326, "Name"="TestMode/TestName") -> ()  [unwired: 9 in, 1 out]
        n197 = property on="Progress" class="Clust (strict)"("Visible"=TRUE) -> ()  [unwired: 2 in, 2 out]
        n198 = property on="Motor" class="Clust (strict)"("Visible"=w323) -> ()  [unwired: 2 in, 2 out]
        n199 = property on="Slider" class="Slide (strict)"("Visible"=w323) -> ()  [unwired: 2 in, 2 out]
        n200 = property on="On/Off" class="Bool (strict)"("Visible"=w323) -> ()  [unwired: 2 in, 2 out]
        n201 = property on="Rev/Fwd" class="Clust (strict)"("Visible"=w323) -> ()  [unwired: 2 in, 2 out]
        n202 = property on="Ring" class="Ring (strict)"("Visible"=w323) -> ()  [unwired: 2 in, 2 out]
      }
      event "Listbox": Double Click {
        n203 = event-data() -> ("PlatMods.Shift"=w331:bool, "Row"=w333:i32)  [unwired: 1 in]
        n204 = case shown="False" w331 {
          tunnel: w333 -> [w337 _]
          tunnel: 1 -> [w336 _]
          frame False {
            n205 = property on="Listbox" class="LstBox (strict)"() -> ("Item Symbols"=w335:i32[])  [unwired: 2 in, 2 out]
            n206 = Replace Array Subset(array=w335, new element=w336, index=w337) -> (w334:i32[])
            n207 = property on="Listbox" class="LstBox (strict)"("Item Symbols"=w334) -> ()  [unwired: 2 in, 2 out]
          }
          frame True {
            w338 = 0 ("Top Row")
            n208 = property on="Listbox" class="LstBox (strict)"() -> ("Number of Rows"=w340:u32)  [unwired: 2 in, 2 out]
            n209 = Initialize Array(0, w340) -> (w339:i32[])
            n210 = property on="Listbox" class="LstBox (strict)"("Top Row"=w338, "Value"=w338, "Item Symbols"=w339) -> ()  [unwired: 2 in, 2 out]
          }
        }
      }
      event "Listbox": Key Down {
        n211 = event-data() -> ("VKey"=w344:T18)  [unwired: 1 in]
        n212 = case shown="\"Left\", \"Right\"" w344 {
          selector: w344 -> [w349 _]
          tunnel: eventvkey."Left" ("VKey") -> [w347 _]
          frame "Left", "Right" {
            n213 = Equal?(x=w347, y=w349) -> (x = y?=w348:bool)
            n214 = Select(t=0, s=w348, f=1) -> (s? t:f=w350:i32)
            n215 = property on="Listbox" class="LstBox (strict)"() -> ("Item Symbols"=w353:i32[])  [unwired: 2 in, 2 out]
            n216 = Replace Array Subset(array=w353, new element=w350, index="Listbox") -> (w352:i32[])
            n217 = property on="Listbox" class="LstBox (strict)"("Item Symbols"=w352) -> ()  [unwired: 2 in, 2 out]
          }
          frame Default {
          }
        }
      }
      event "DB Camera Config": Value Change {
        n218 = event-data() -> ("NewVal"=w357:bool)  [unwired: 1 in]
        n219 = case shown="False" w357 {
          tunnel: w356 -> [w366 _]
          tunnel: [w359 w377] -> w355
          tunnel: w354 -> [w358 w377]
          frame False {
            w373 = "Camera"
            w376 = FALSE ("Visible")
            n220 = local read "Camera Settings"() -> (w365:T1)
            n221 = Index Array(array=w366) -> (element=w369:cluster{string[]})  [unwired: 1 in]
            n222 = Unbundle(w365) -> ("Frate Rate"=w364:i32, "Compression"=w363:i32, "Size"=w367:u16)
            n223 = Unbundle(w369) -> (w368:string[])
            n224 = Index Array(array=w368, index=w367) -> (element=w362:string)
            n225 = call-poly <vilib>:"Write Key.vi"("section"=w373, "value"=w362, "key"="Size", "refnum"=w358) -> ("refnum out"=w375:T17)  [unwired: 2 in, 5 out]
            n226 = call-poly <vilib>:"Write Key.vi"("section"=w373, "value"=w364, "key"="FrameRate", "refnum"=w375) -> ("refnum out"=w374:T17)  [unwired: 1 in, 6 out]
            n227 = property on="Camera Settings" class="Clust (strict)"("Visible"=w376) -> ()  [unwired: 2 in, 2 out]
            n228 = local write "DB Camera Config"(w376) -> ()
            n229 = call-poly <vilib>:"Write Key.vi"("section"=w373, "value"=w363, "key"="Compression", "refnum"=w374) -> ("refnum out"=w360:T17)  [unwired: 1 in, 6 out]
            n230 = call <vilib>:"Close Config Data.vi"("refnum"=w360) -> ("file path"=w361:path)  [unwired: 2 in, 8 out]
            n231 = call <vilib>:"Open Config Data.vi"("configuration file path"=w361) -> ("refnum"=w359:T17)  [unwired: 8 in, 2 out]
          }
          frame True {
            n232 = property on="Camera Settings" class="Clust (strict)"("Visible"=TRUE) -> ()  [unwired: 2 in, 2 out]
          }
        }
      }
      event "Camera Settings": Value Change {
        n233 = event-data() -> ("NewVal"=w390:T1)  [unwired: 1 in]
        n234 = Index Array(array=w386) -> (element=w385:cluster{string[]})  [unwired: 1 in]
        n235 = Unbundle(w390) -> ("Frate Rate"=w381:i32, "Compression"=w380:i32, "Size"=w383:u16)
        n236 = Unbundle(w385) -> (w384:string[])
        n237 = Index Array(array=w384, index=w383) -> (element=w382:string)
        n238 = Format Into String(format string="%s   %dfps   %d%%", w382, w381, w380) -> (resulting string=w387:string)  [unwired: 2 in, 1 out]
        n239 = Build Array(w387) -> (w388:string[])
        n240 = property on="DB Camera Config" class="Bool (strict)"("Strings [4]"=w388) -> ()  [unwired: 2 in, 2 out]
      }
      event "Motor.Enable": Value Change {
        n241 = event-data() -> ("NewVal"=w396:bool)  [unwired: 1 in]
        n242 = Unbundle("Motor") -> ("Value"=w395:dbl)  [unwired: 1 out]
        n243 = Select(t=w395, s=w396, f=0.0) -> (s? t:f=w393:dbl)
        n244 = call <vilib>:"NT Write Number.vi"("Numeric"=w393, "Name"=w392) -> ()  [unwired: 9 in, 1 out]
      }
      event "Slider": Value Change {
        n245 = event-data() -> ("NewVal"=w399:dbl)  [unwired: 1 in]
        n246 = call <vilib>:"NT Write Number.vi"("Numeric"=w399, "Name"=w400) -> ()  [unwired: 9 in, 1 out]
      }
      event "On/Off": Value Change {
        n247 = event-data() -> ("NewVal"=w404:bool)  [unwired: 1 in]
        n248 = Boolean To (0,1)(Boolean=w404) -> (0, 1=w403:i16)
        n249 = call <vilib>:"NT Write Number.vi"("Numeric"=w403, "Name"=w402) -> ()  [unwired: 9 in, 1 out]
      }
      event "Rev/Fwd": Value Change {
        n250 = event-data() -> ("NewVal.Forward"=w412:bool, "NewVal.Reverse"=w411:bool)  [unwired: 1 in]
        n251 = Boolean To (0,1)(Boolean=w412) -> (0, 1=w408:i16)
        n252 = Boolean To (0,1)(Boolean=w411) -> (0, 1=w410:i16)
        n253 = Negate(x=w410) -> (-x=w409:i16)
        n254 = Add(x=w408, y=w409) -> (x+y=w407:i16)
        n255 = call <vilib>:"NT Write Number.vi"("Numeric"=w407, "Name"=w406) -> ()  [unwired: 9 in, 1 out]
      }
      event "Ring": Value Change {
        n256 = event-data() -> ("NewVal"=w416:u16)  [unwired: 1 in]
        n257 = property on="Ring" class="Ring (strict)"() -> ("Strings []"=w417:string[])  [unwired: 2 in, 2 out]
        n258 = Index Array(array=w417, index=w416) -> (element=w415:string)
        n259 = call <vilib>:"NT Write String.vi"("String"=w415, "Name"=w414) -> ()  [unwired: 9 in, 1 out]
      }
    }
  }
  n260 = Index Array(array=w19) -> (element=w20:cluster{string[]})  [unwired: 1 in]
  n261 = Unbundle(w20) -> (w18:string[])
  n262 = Match First String(2:w18, 3:w17) -> (0:w16:i32)  [unwired: 1 out]
  n263 = disable-structure shown="Disabled" {
    disable-tunnel: [w419 _] -> w6
    frame Disabled {
      n264 = call <vilib>:"SD Read Number.vi"("Name"="Front Shooter Feedback") -> ("Numeric"=w419:dbl)  [unwired: 8 in, 2 out]
    }
    frame Enabled {
    }
  }
  "Front Shooter Feedback" <- w6
  n265 = disable-structure shown="Disabled" {
    disable-tunnel: [w421 _] -> w4
    frame Disabled {
      n266 = call <vilib>:"SD Read Number.vi"("Name"="Back Shooter Feedback") -> ("Numeric"=w421:dbl)  [unwired: 8 in, 2 out]
    }
    frame Enabled {
    }
  }
  "Back Shooter Feedback" <- w4
  n267 = Bundle("value"=w22, "value"=w21, "index"=w16) -> (w10:cluster{"value":i32, "value":i32, "index":i32})  [unwired: 1 out]
  n268 = disable-structure shown="Disabled" {
    disable-tunnel: [w423 _] -> w3
    frame Disabled {
      n269 = call <vilib>:"SD Read Number.vi"("Name"="Ball Screw Feedback") -> ("Numeric"=w423:dbl)  [unwired: 8 in, 2 out]
    }
    frame Enabled {
    }
  }
  "Ball Screw \nFeedback" <- w3
  n270 = property on="On/Off" class="Bool (strict)"("Visible"=w33) -> ()  [unwired: 2 in, 2 out]
  n271 = property on="Motor" class="Clust (strict)"("Visible"=w33) -> ()  [unwired: 2 in, 2 out]
  n272 = property on="Progress" class="Clust (strict)"("Visible"=w33) -> ()  [unwired: 2 in, 2 out]
  n273 = property on="Ring" class="Ring (strict)"("Visible"=w33) -> ()  [unwired: 2 in, 2 out]
  n274 = property on="Camera Settings" class="Clust (strict)"("Val(Sgnl)"=w10) -> ()  [unwired: 2 in, 2 out]
  n275 = property on="Rev/Fwd" class="Clust (strict)"("Visible"=w33) -> ()  [unwired: 2 in, 2 out]
  n276 = property on="Camera Settings" class="Clust (strict)"("Visible"=w33) -> ()  [unwired: 2 in, 2 out]
  n277 = local write "DB Camera Config"(w33) -> ()
  n278 = disable-structure shown="Disabled" {
    disable-tunnel: "Ball Screw Angle" -> [w425 _]
    frame Disabled {
      n279 = call <vilib>:"SD Write Number.vi"("Numeric"=w425, "Name"="Ball Screw Angle") -> ()  [unwired: 8 in, 2 out]
    }
    frame Enabled {
    }
  }
  n280 = disable-structure shown="Disabled" {
    disable-tunnel: "Back Shooter Speed" -> [w427 _]
    frame Disabled {
      n281 = call <vilib>:"SD Write Number.vi"("Numeric"=w427, "Name"="Back Shooter Speed") -> ()  [unwired: 8 in, 2 out]
    }
    frame Enabled {
    }
  }
  n282 = disable-structure shown="Disabled" {
    disable-tunnel: "Front Shooter Speed" -> [w429 _]
    frame Disabled {
      n283 = call <vilib>:"SD Write Number.vi"("Numeric"=w429, "Name"="Front Shooter Speed") -> ()  [unwired: 8 in, 2 out]
    }
    frame Enabled {
    }
  }
